vi "ComputeCOM.vi"(3 "tracker":u64) -> (0 "Center of mass":cluster{"comX":sgl, "comY":sgl}, 1 "tracker":u64)   [LabVIEW 2011]
uses:
  cudatrack-debug.dll
panel:
  in  "comX":sgl
  in  "comY":sgl
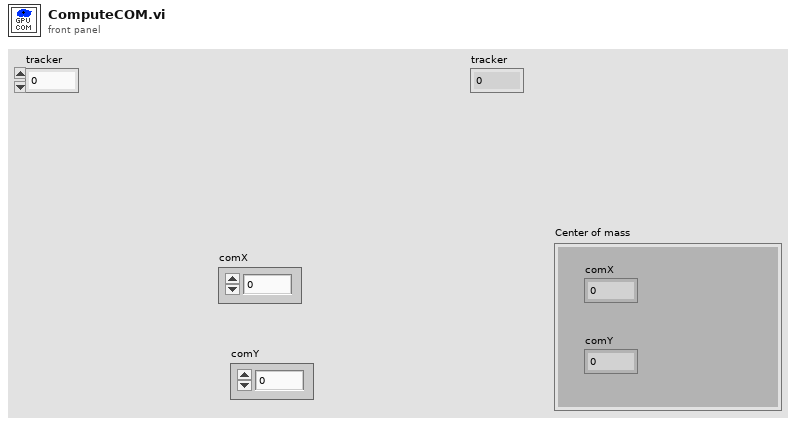
[diagram p1: front panel]
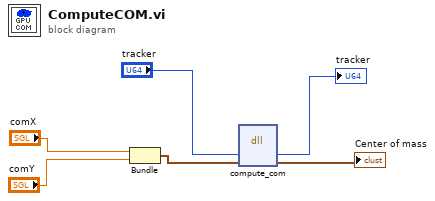
[diagram p0: block diagram]
diagram:
  n1 = Bundle("comX"="comX", "comY"="comY") -> (w4:cluster{"comX":sgl, "comY":sgl})  [unwired: 1 in]
  n2 = dll-call lib="D:/jcnossen1/cudaqi-tracker/cudatrack/cudatrack-debug.dll" fn="compute_com"("tracker"="tracker", "position"=w4) -> ("tracker"=→"tracker":u64, "position"=→"Center of mass":cluster{"comX":sgl, "comY":sgl})  [unwired: 4 in, 2 out]
